vi "Set Board Number.vi"(8 "error in (no error)":errorcluster, 10 "Board Number":i32 max=256 step=1, 11 "Pulseblaster in":refnum<class "Slave_Pulseblaster.lvclass">) -> (0 "error out":errorcluster, 3 "Pulseblaster out":refnum<class "Slave_Pulseblaster.lvclass">)   [LabVIEW 2013, in "Slave_Pulseblaster.lvclass"]
uses:
  Slave_Pulseblaster.lvclass
  Slave_Pulseblaster.lvclass/Slave_Pulseblaster.ctl
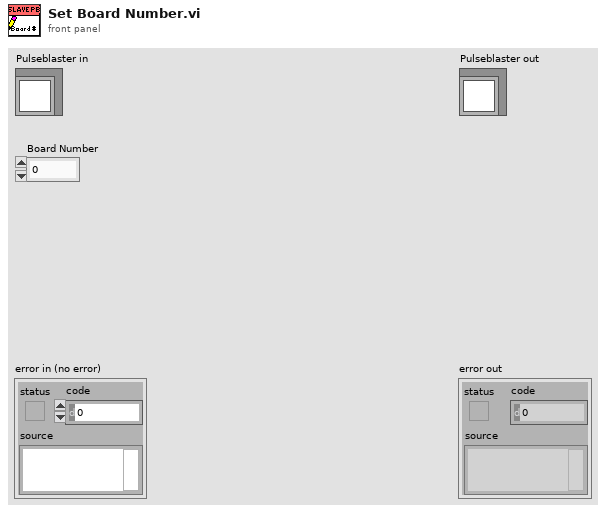
[diagram p1: front panel]
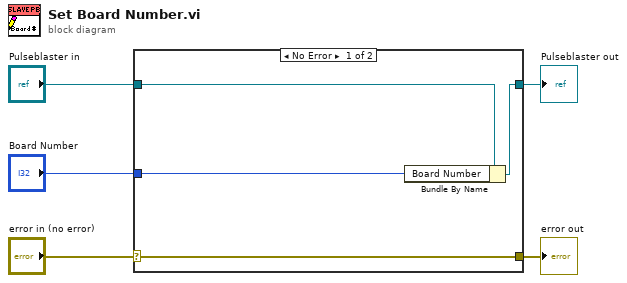
[diagram p0: block diagram]
diagram:
  n1 = case shown="No Error" "error in (no error)" {
    selector: "error in (no error)" -> [w9 w10]
    tunnel: [w9 w10] -> w4
    tunnel: [w7 w11] -> w2
    tunnel: "Pulseblaster in" -> [w8 w11]
    tunnel: "Board Number" -> [w6 _]
    frame No Error {
      n2 = Bundle By Name(cluster=w8, "Board Number"=w6) -> (w7:refnum<class "Slave_Pulseblaster.lvclass">)
    }
    frame Error {
    }
  }
  "error out" <- w4
  "Pulseblaster out" <- w2
